vi "Insert RPM Data.vi"(6 "Available Tests":T1, 7 "Raw":dbl[](array[numeric]), 9 "Numeric":i32, 10 "Data Out in":waveform(dbl)[](array[waveform]), 11 "Pulsed RPM Capture":bool) -> (0 "error out":errorcluster, 1 "Measurements":string, 2 "Header":string, 3 "Data Out out":string[][](array[string]), 5 "Waveform":waveform(dbl))   [LabVIEW 2017]
uses:
  Controls/Available Tests.ctl
  <vilib>/Analysis/baseanly.llb/Mean (DBL).vi
  <vilib>/Analysis/NI_AALBase.lvlib
panel:
  out "Waveform 2":waveform(dbl)
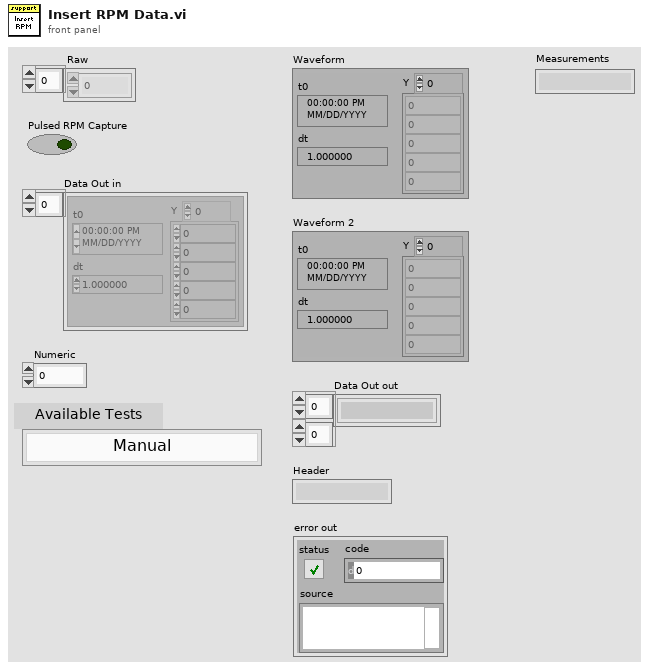
[diagram p1: front panel]
types:
  T1 = typedef "Available Tests.ctl" = enum16{"Manual", "EFX Brake Torque", "Generator Torque", "EFX Brake Thermal", "Generator Thermal", "Pulsed RPM", "AMT Brake Torque", "Bike Brake Torque", "AMT Brake Thermal", "Bike Brake Thermal"}
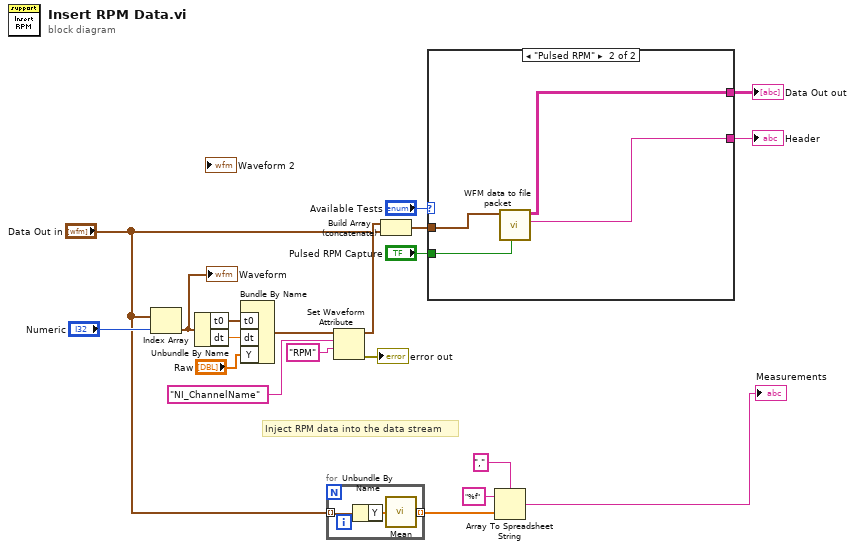
[diagram p0: block diagram]
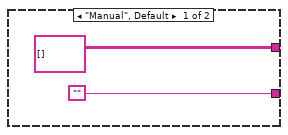
[diagram p2: hidden frame]
diagram:
  # "Inject RPM data into the data stream"
  n1 = Index Array(array="Data Out in", index="Numeric") -> (element=w6:waveform(dbl))
  "Waveform" <- w6
  n2 = Unbundle By Name(w6) -> ("t0"=w8:timestamp, "dt"=w9:dbl)
  n3 = Bundle By Name("t0"=w8, "dt"=w9, "Y"="Raw") -> (w12:waveform(dbl))  [unwired: 1 in]
  n4 = for {
    tunnel: "Data Out in" -> [w23] mode=indexing
    tunnel: [w21] -> w4 mode=indexing
    n5 = Unbundle By Name(w23) -> ("Y"=w22:dbl[])
    n6 = call-poly <vilib>:"Mean.vi"("X"=w22) -> ("mean"=w21:dbl)  [unwired: 1 out]
  }
  n7 = Set Waveform Attribute(5:"RPM", 6:"NI_ChannelName" ("name"), 7:w12) -> (0:→"error out":errorcluster, 3:w16:waveform(dbl))  [unwired: 1 in, 1 out]
  n8 = Build Array (concatenate)(w16, "Data Out in") -> (w10:waveform(dbl)[])
  n9 = case shown="\"Pulsed RPM\"" "Available Tests" {
    tunnel: w10 -> [_ w29]
    tunnel: [string[][] [] ("appended array") w28] -> w11
    tunnel: ["" w27] -> w18
    tunnel: "Pulsed RPM Capture" -> [_ w26]
    frame "Manual", Default {
    }
    frame "Pulsed RPM" {
      n10 = call "WFM data to file packet.vi"("Save RPM Data"=w26, "WFM Data In"=w29) -> ("Header"=w27:string, "Data Out"=w28:string[][])  [unwired: 8 in]
    }
  }
  "Header" <- w18
  "Data Out out" <- w11
  n11 = Array To Spreadsheet String(delimiter (Tab)=",", array=w4, 3:"%f" ("format string")) -> (spreadsheet string=→"Measurements":string)
